vi "Read Timing Path.vi"(8 "error in (no error)":errorcluster, 11 "Dispense in":refnum<class "Dispense.lvclass">) -> (0 "error out":errorcluster, 2 "Timing Path":path, 3 "Dispense out":refnum<class "Dispense.lvclass">)   [LabVIEW 2016, in "Dispense.lvclass"]
uses:
  Dispense.lvclass
  Dispense.lvclass/Dispense.ctl
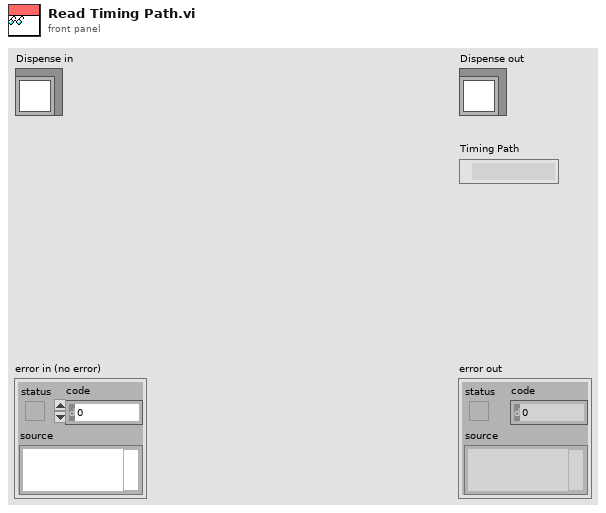
[diagram p1: front panel]
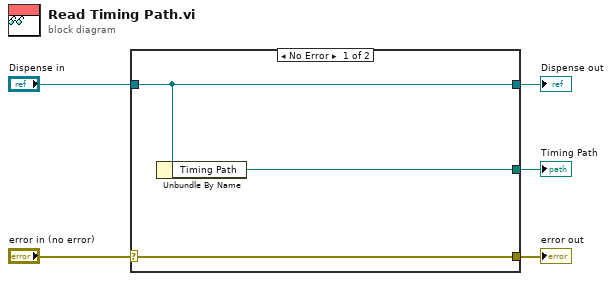
[diagram p0: block diagram]
diagram:
  n1 = case shown="No Error" "error in (no error)" {
    selector: "error in (no error)" -> [w8 w9]
    tunnel: [w8 w9] -> w4
    tunnel: [w7 w10] -> w2
    tunnel: "Dispense in" -> [w7 w10]
    tunnel: [w6 _] -> w1
    frame No Error {
      n2 = Unbundle By Name(w7) -> ("Timing Path"=w6:path)
    }
    frame Error {
    }
  }
  "error out" <- w4
  "Dispense out" <- w2
  "Timing Path" <- w1
